vi "Fases_U_W_Corriente.vi"(0 "Amplitud Corrientes":fxp<+,32,0>, 1 "U-V":fxp<+/-,17,3>, 4 "V-W":fxp<+/-,17,3>, 5 "W-U":fxp<+/-,17,3>, 7 "Cluster Diferencia de Voltajes":T1, 8 "Polaridad L-K en U?":bool, 9 "Polaridad L-K en W?":bool) -> (21 "Pulsos Corriente U":fxp<+/-,34,2>, 25 "Pulsos Corriente W":fxp<+/-,34,2>)   [LabVIEW 2020]
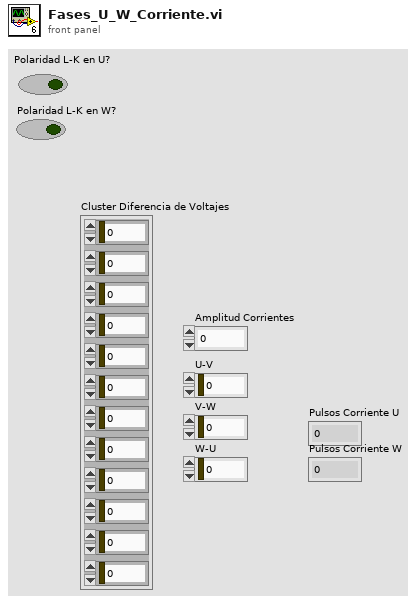
[diagram p1: front panel]
types:
  T1 = cluster{fxp<+/-,17,3>, fxp<+/-,17,3>, fxp<+/-,17,3>, fxp<+/-,17,3>, fxp<+/-,17,3>, fxp<+/-,17,3>, fxp<+/-,17,3>, fxp<+/-,17,3>, fxp<+/-,17,3>, fxp<+/-,17,3>, fxp<+/-,17,3>, fxp<+/-,17,3>}
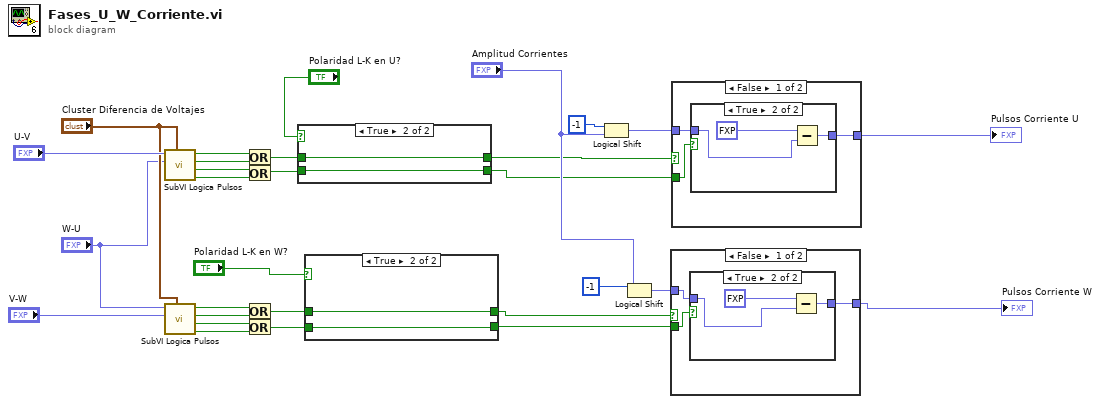
[diagram p0: block diagram]
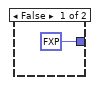
[diagram p4: hidden frame]
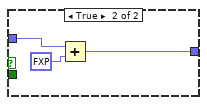
[diagram p5: hidden frame]
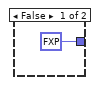
[diagram p6: hidden frame]
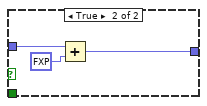
[diagram p7: hidden frame]
diagram:
  n1 = call "SubVI Logica Pulsos.vi"("Cluster Diferencia de Voltajes"="Cluster Diferencia de Voltajes", "fase-fase 2"="W-U", "fase-fase 1"="U-V") -> ("Segundo Pulso Negativo"=w7:bool, "Primer Pulso Negativo"=w8:bool, "Segundo Pulso Positivo"=w9:bool, "Primer Pulso Positivo"=w10:bool)  [unwired: 5 in]
  n2 = call "SubVI Logica Pulsos.vi"("Cluster Diferencia de Voltajes"="Cluster Diferencia de Voltajes", "fase-fase 2"="V-W", "fase-fase 1"="W-U") -> ("Segundo Pulso Negativo"=w3:bool, "Primer Pulso Negativo"=w4:bool, "Segundo Pulso Positivo"=w5:bool, "Primer Pulso Positivo"=w6:bool)  [unwired: 5 in]
  n3 = Or(x=w10, y=w9) -> (x .or. y?=w22:bool)
  n4 = Or(x=w8, y=w7) -> (x .or. y?=w25:bool)
  n5 = Or(x=w6, y=w5) -> (x .or. y?=w26:bool)
  n6 = Or(x=w4, y=w3) -> (x .or. y?=w27:bool)
  n7 = case shown="True" "Polaridad L-K en U?" {
    tunnel: w22 -> [w31 w33]
    tunnel: [w30 w33] -> w23
    tunnel: [w31 w32] -> w24
    tunnel: w25 -> [w30 w32]
    frame False {
    }
    frame True {
    }
  }
  n8 = case shown="True" "Polaridad L-K en W?" {
    tunnel: w26 -> [w35 w37]
    tunnel: [w34 w37] -> w14
    tunnel: [w35 w36] -> w13
    tunnel: w27 -> [w34 w36]
    frame False {
    }
    frame True {
    }
  }
  n9 = Logical Shift(y=i16 -1, x="Amplitud Corrientes") -> (x << y=w16:fxp<+,32,0>)
  n10 = Logical Shift(y=i16 -1, x="Amplitud Corrientes") -> (x << y=w17:fxp<+,32,0>)
  n11 = case shown="False" w14 {
    tunnel: w17 -> [w40 w46]
    tunnel: [w39 w45] -> w1
    tunnel: w13 -> [w38 _]
    frame False {
      n12 = case shown="True" w38 {
        tunnel: w40 -> [_ w42]
        tunnel: [fxp<+/-,33,1> 0.5 w44] -> w39
        frame False {
        }
        frame True {
          n13 = Subtract(x=fxp<+,32,0> 0.5 ("duty cycle (periods)"), y=w42) -> (x-y=w44:fxp<+/-,33,1>)
        }
      }
    }
    frame True {
      n14 = Add(x=w46, y=fxp<+,32,0> 0.5 ("duty cycle (periods)")) -> (x+y=w45:fxp<+,33,1>)
    }
  }
  "Pulsos Corriente W" <- w1
  n15 = case shown="False" w23 {
    tunnel: w16 -> [w49 w56]
    tunnel: [w48 w55] -> w2
    tunnel: w24 -> [w50 _]
    frame False {
      n16 = case shown="True" w50 {
        tunnel: w49 -> [_ w52]
        tunnel: [fxp<+/-,33,1> 0.5 w54] -> w48
        frame False {
        }
        frame True {
          n17 = Subtract(x=fxp<+,32,0> 0.5 ("duty cycle (periods)"), y=w52) -> (x-y=w54:fxp<+/-,33,1>)
        }
      }
    }
    frame True {
      n18 = Add(x=w56, y=fxp<+,32,0> 0.5 ("duty cycle (periods)")) -> (x+y=w55:fxp<+,33,1>)
    }
  }
  "Pulsos Corriente U" <- w2
